vi "__getRoomMap.vi"(11 "Room-API in":refnum<class "Room-API.lvclass">) -> (2 "room_map":map{string, T1}(c390), 3 "Room-API out":refnum<class "Room-API.lvclass">)   [LabVIEW 2020, in "Room-API.lvclass"]
uses:
  Room-API.lvclass
  Single Room.ctl
  Room-API.lvclass/Room-API.ctl
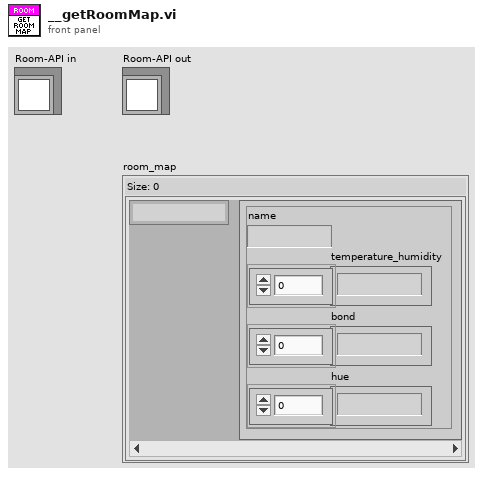
[diagram p1: front panel]
types:
  T1 = typedef "Room-API.lvclass/Single Room.ctl" = cluster{"name":string, "temperature_humidity":string[], "bond":string[], "hue":string[]}
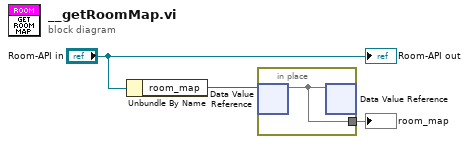
[diagram p0: block diagram]
diagram:
  n1 = Unbundle By Name("Room-API in") -> ("room_map"=w2:refnum<data-value>)
  n2 = in-place {
    in-place-border: [w4] -> w3
    n3 = in-place-dvr #1(w2) -> (w4:map{string, T1})  [unwired: 1 out]
    n4 = in-place-dvr #1(w4) -> ()  [unwired: 2 out]
  }
  "room_map" <- w3
  "Room-API out" <- "Room-API in"
